vi "testbytestrings.vi"() -> ()   [LabVIEW 2014]
panel:
  in  "subset length":i32=10
  out "Subset String":string
  out "String as byte array Subset":u8[](array[numeric])
  out "String as boolean array":bool[](array[boolean])
  out "String as byte array":u8[](array[numeric])
  in  "String":string
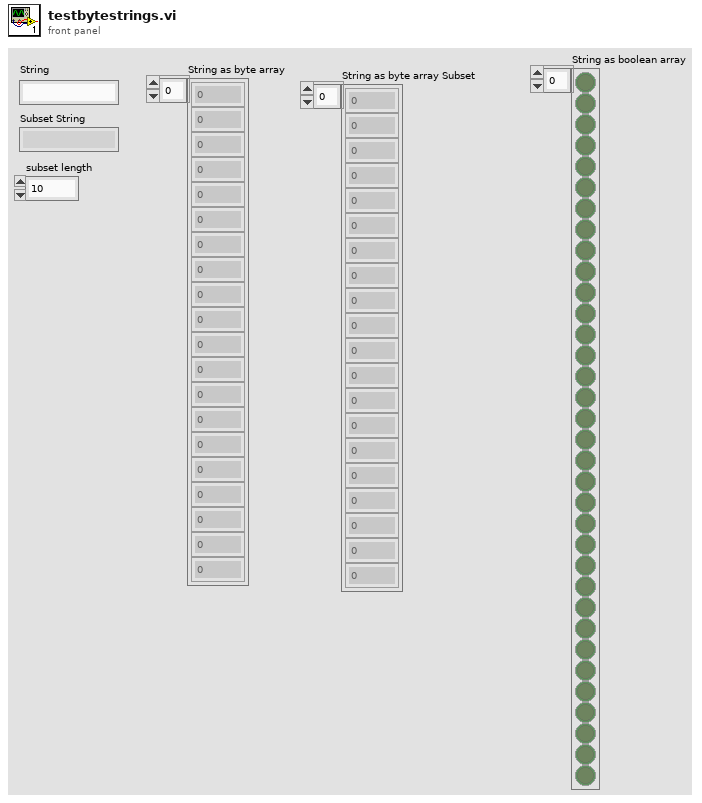
[diagram p1: front panel]
types:
  T1 = enum16{"big-endian, network order", "native, host order", "little-endian"}
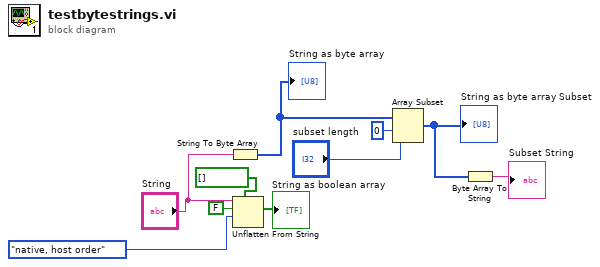
[diagram p0: block diagram]
diagram:
  n1 = String To Byte Array(string="String") -> (unsigned byte array=w5:u8[])
  "String as byte array" <- w5
  n2 = Unflatten From String(type=bool[] [], binary string="String", data includes array or string size? (T)=FALSE, byte order (0:big-endian, network order)=T1."native, host order") -> (value=→"String as boolean array":bool[])  [unwired: 1 in, 2 out]
  n3 = Array Subset(array=w5, index=0, length="subset length") -> (w2:u8[])
  "String as byte array Subset" <- w2
  n4 = Byte Array To String(unsigned byte array=w2) -> (string=→"Subset String":string)
